vi "Launch cRIO-CO2 Actor.vi"(8 "error in (no error)":errorcluster, 11 "Refs for Debuging":T1) -> (0 "error out":errorcluster, 3 "Caller-To-Actor Enqueuer":refnum<class "Message Enqueuer.lvclass">)   [LabVIEW 2015, in "cRIO-Carbondioxide.lvlib" / "cRIO-CO2.lvlib" / "cRIO-CO2.lvclass"]
uses:
  cRIO-CO2.lvclass
  <vilib>/ActorFramework/Message Enqueuer/Message Enqueuer.lvclass
  Debugger.ctl
  <vilib>/ActorFramework/Actor/Actor.lvclass
  cRIO-CO2.lvclass/cRIO-CO2.ctl
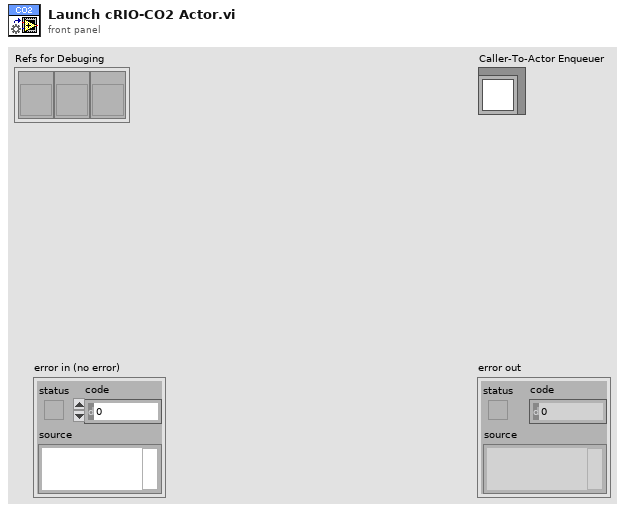
[diagram p1: front panel]
types:
  T1 = typedef "cRIO-Carbondioxide.lvlib/cRIO-CO2.lvlib/cRIO-CO2.lvclass/Debugger.ctl" = cluster{"Log Ref":refnum<vi>, "Debugger Graph Chart Ref":refnum<vi>, "Debug Rng Ref":refnum<vi>}
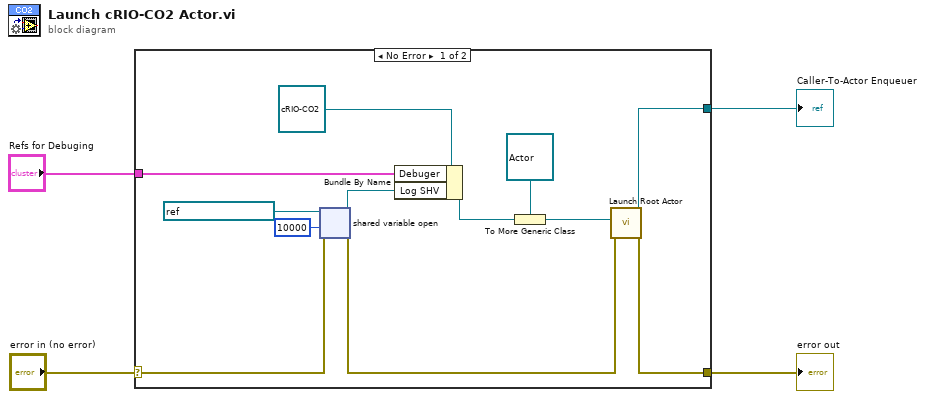
[diagram p0: block diagram]
diagram:
  n1 = case shown="No Error" "error in (no error)" {
    selector: "error in (no error)" -> [w12 w17]
    tunnel: [w16 w17] -> w3
    tunnel: [w15 _] -> w2
    tunnel: "Refs for Debuging" -> [w10 _]
    frame No Error {
      n2 = shared-variable-open(refnum<k21> "ni.var.psp://cRIO-Carbondioxide/AMS Gas SHV/Log" ("shared variable refnum in"), w12, 10000 ("timeout ms")) -> (w11:refnum<k21>, w8:errorcluster)  [unwired: 1 in]
      n3 = Bundle By Name(cluster=refnum<class "cRIO-CO2.lvclass"> refnum ("cRIO-CO2 in"), "Debuger"=w10, "Log SHV"=w11) -> (w7:refnum<class "cRIO-CO2.lvclass">)
      n4 = To More Generic Class(target class=refnum<class "Actor.lvclass"> refnum ("Actor"), reference=w7) -> (generic class reference=w5:refnum<class "Actor.lvclass">)
      n5 = call <vilib>:"Launch Root Actor.vi"("error in (no error)"=w8, "Actor"=w5) -> ("error out"=w16:errorcluster, "Actor's Enqueuer"=w15:refnum<class "Message Enqueuer.lvclass">)  [unwired: 8 in]
    }
    frame Error {
    }
  }
  "error out" <- w3
  "Caller-To-Actor Enqueuer" <- w2
